vi "Grating Position to Wavelength.vi"(5 "grating index (0)":u8, 7 "turret index (0)":u8, 8 "error in (no error)":errorcluster, 10 "grating position":i32, 11 "SOL MS in":refnum<class "PL SOL Instruments MS.lvclass">) -> (0 "error out":errorcluster, 2 "wavelength, nm":dbl, 3 "SOL MS out":refnum<class "PL SOL Instruments MS.lvclass">)   [LabVIEW 2015, in "PL SOL Instruments MS.lvclass"]
doc: "Converts <b>grating position</b> of the specified <b>grating</b> of the specified <b>turret</b> to <b>wavelength</b>."
uses:
  PL SOL Instruments MS.lvclass
  PL SOL Instruments MS.lvclass/PL SOL Instruments MS.ctl
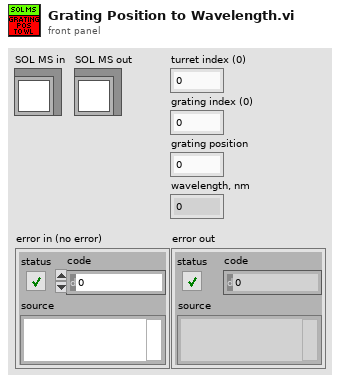
[diagram p1: front panel]
types:
  T1 = cluster{"name":string, "step timeout, ms":u32, "reset timeout, ms":u32, "gratings":cluster{"name":string, "step timeout, ms":u32, "reset timeout, ms":u32, "turret position":i32, "reset position":i32, "max position":i32, "backlash distance":i32, "step size, rad":dbl, "groove density, g/mm":dbl, "theta2, rad":dbl, "blaze wavelength, nm":dbl, "focal length, cm":dbl, "manual change":bool, "manual change position":i32}[], "current grating":cluster{"index":u8, "position":i32}}[]
  T2 = cluster{"name":string, "step timeout, ms":u32, "reset timeout, ms":u32, "gratings":cluster{"name":string, "step timeout, ms":u32, "reset timeout, ms":u32, "turret position":i32, "reset position":i32, "max position":i32, "backlash distance":i32, "step size, rad":dbl, "groove density, g/mm":dbl, "theta2, rad":dbl, "blaze wavelength, nm":dbl, "focal length, cm":dbl, "manual change":bool, "manual change position":i32}[], "current grating":cluster{"index":u8, "position":i32}}
  T3 = cluster{"name":string, "step timeout, ms":u32, "reset timeout, ms":u32, "turret position":i32, "reset position":i32, "max position":i32, "backlash distance":i32, "step size, rad":dbl, "groove density, g/mm":dbl, "theta2, rad":dbl, "blaze wavelength, nm":dbl, "focal length, cm":dbl, "manual change":bool, "manual change position":i32}[]
  T4 = cluster{"name":string, "step timeout, ms":u32, "reset timeout, ms":u32, "turret position":i32, "reset position":i32, "max position":i32, "backlash distance":i32, "step size, rad":dbl, "groove density, g/mm":dbl, "theta2, rad":dbl, "blaze wavelength, nm":dbl, "focal length, cm":dbl, "manual change":bool, "manual change position":i32}
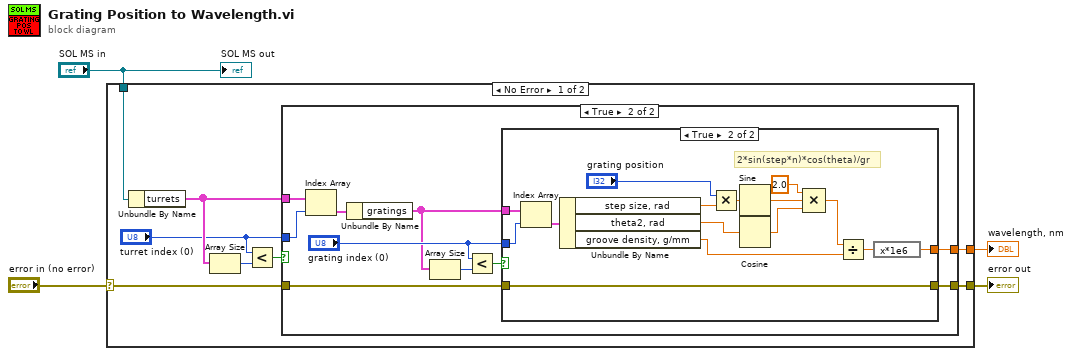
[diagram p0: block diagram]
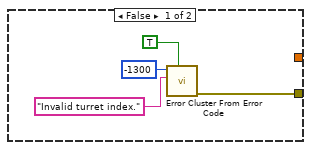
[diagram p2: hidden frame]
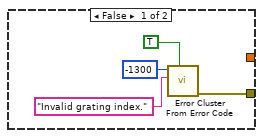
[diagram p3: hidden frame]
diagram:
  n1 = case shown="No Error" "error in (no error)" {
    selector: "error in (no error)" -> [w6 w46]
    tunnel: "SOL MS in" -> [w12 _]
    tunnel: [w11 _] -> w3
    tunnel: [w7 w46] -> w1
    frame No Error {
      n2 = Unbundle By Name(w12) -> ("turrets"=w10:T1)
      n3 = Array Size(array=w10) -> (size(s)=w9:i32)
      n4 = Less?(x="turret index (0)", y=w9) -> (x < y?=w8:bool)
      n5 = case shown="True" w8 {
        tunnel: w10 -> [_ w26]
        tunnel: [_ w24] -> w11
        tunnel: [w13 w19] -> w7
        tunnel: w6 -> [_ w17]
        tunnel: "turret index (0)" -> [_ w18]
        frame False {
          n6 = call <vilib>:"Error Cluster From Error Code.vi"("show call chain? (False)"=TRUE, "error message (\"\")"="Invalid turret index." ("error message (\"\")"), "error code (0)"=-1300) -> ("error out"=w13:errorcluster)  [unwired: 6 in]
        }
        frame True {
          n7 = Index Array(array=w26, index=w18) -> (element=w25:T2)
          n8 = Unbundle By Name(w25) -> ("gratings"=w21:T3)
          n9 = Array Size(array=w21) -> (size(s)=w23:i32)
          n10 = Less?(x="grating index (0)", y=w23) -> (x < y?=w20:bool)
          n11 = case shown="True" w20 {
            tunnel: w21 -> [_ w45]
            tunnel: "grating index (0)" -> [_ w44]
            tunnel: [_ w32] -> w24
            tunnel: [w27 w31] -> w19
            tunnel: w17 -> [_ w31]
            frame False {
              n12 = call <vilib>:"Error Cluster From Error Code.vi"("show call chain? (False)"=TRUE, "error message (\"\")"="Invalid grating index." ("error message (\"\")"), "error code (0)"=-1300) -> ("error out"=w27:errorcluster)  [unwired: 6 in]
            }
            frame True {
              # "2*sin(step*n)*cos(theta)/gr"
              n13 = Index Array(array=w45, index=w44) -> (element=w43:T4)
              n14 = Unbundle By Name(w43) -> ("step size, rad"=w36:dbl, "theta2, rad"=w34:dbl, "groove density, g/mm"=w33:dbl)
              n15 = Multiply(x="grating position", y=w36) -> (x*y=w42:dbl)
              n16 = Sine(x=w42) -> (sin(x)=w41:dbl)
              n17 = Cosine(x=w34) -> (cos(x)=w39:dbl)
              n18 = Compound Arithmetic op=MULTIPLY(2.0 ("value"), w41, w39) -> (w38:dbl)
              n19 = Divide(x=w38, y=w33) -> (x/y=w37:dbl)
              n20 = expression code="x*1e6"(w37) -> (w32:dbl)
            }
          }
        }
      }
    }
    frame Error {
    }
  }
  "wavelength, nm" <- w3
  "error out" <- w1
  "SOL MS out" <- "SOL MS in"
